vi "overlay_axis_particle(subVI).vi"(8 "error in (no error)":errorcluster, 9 "filtred & calibrated image":T1, 10 "view image":T1) -> (0 "error out":errorcluster, 1 "Particle Reports (Real-World)":T2(array[cluster]) {"Orientation" format="%.2f"; "Dimensions"."Height" format="%.2f"; "Dimensions"."Width" format="%.2f"; "Center of Mass"."Y" format="%.2f"; "Center of Mass"."X" format="%.2f"; "Bounding Rect"."Bottom" format="%.2f"; "Bounding Rect"."Right" format="%.2f"; "Bounding Rect"."Top" format="%.2f"; "Bounding Rect"."Left" format="%.2f"; "Number of Holes" format="%.2f"; "Area" format="%.2f"}, 2 "number of particle":i32, 3 "Image Out":T1)   [LabVIEW 2020]
uses:
  <vilib>/vision/Image Controls.llb/IMAQ Image.ctl
  <vilib>/vision/NI_Vision_Development_Module.lvlib
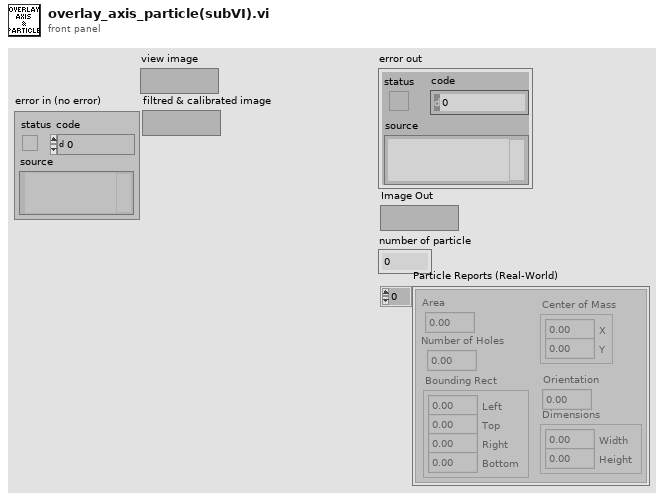
[diagram p1: front panel]
types:
  T1 = typedef "IMAQ Image.ctl" = refnum<image>
  T2 = cluster{"Area":dbl, "Number of Holes":dbl, "Bounding Rect":cluster{"Left":dbl, "Top":dbl, "Right":dbl, "Bottom":dbl}, "Center of Mass":cluster{"X":dbl, "Y":dbl}, "Orientation":dbl, "Dimensions":cluster{"Width":dbl, "Height":dbl}}[]
  T3 = cluster{"Origin Pixel":cluster{"X":sgl, "Y":sgl}, "Angle Relative to Horizontal (deg)":sgl, "Axis Reference":u32}
  T4 = cluster{"Origin Pixel":cluster{"X":sgl, "Y":sgl}, "Angle Relative to Horizontal (deg)":sgl, "X Axis Pixel":cluster{"X":sgl, "Y":sgl}, "Axis Reference":u32}
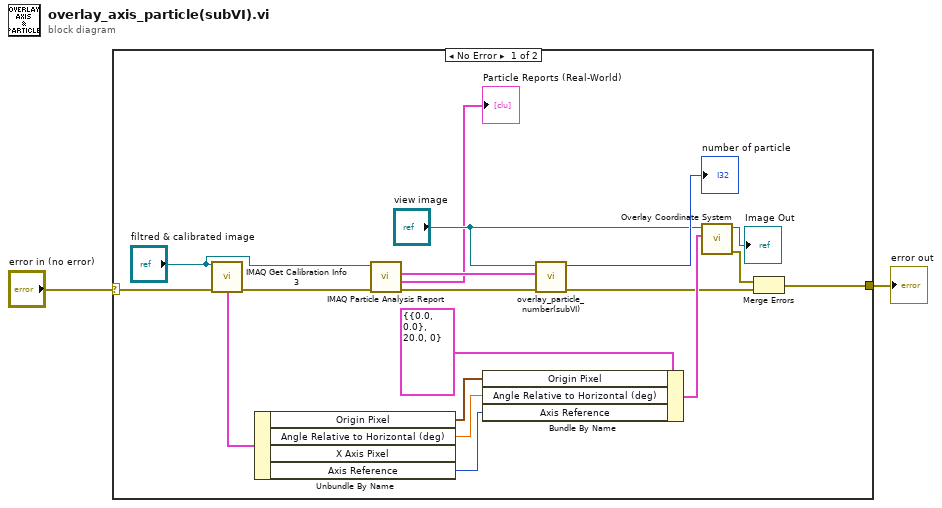
[diagram p0: block diagram]
diagram:
  n1 = case shown="No Error" "error in (no error)" {
    selector: "error in (no error)" -> [w13 w21]
    tunnel: [w15 w21] -> w2
    frame No Error {
      n2 = call "IMAQ Get Calibration Info 3"("Calibration Template Image"="filtred & calibrated image", "error in (no error)"=w13) -> ("Calibration Axis Info"=w8:T4, "error out"=w11:errorcluster)  [unwired: 5 in, 7 out]
      n3 = Unbundle By Name(w8) -> ("Origin Pixel"=w6:cluster{"X":sgl, "Y":sgl}, "Angle Relative to Horizontal (deg)"=w5:sgl, "Axis Reference"=w7:u32)  [unwired: 1 out]
      n4 = call "IMAQ Particle Analysis Report"("error in (no error)"=w11, "Image"="filtred & calibrated image") -> ("error out"=w10:errorcluster, "Particle Reports (Real-World)"=→"Particle Reports (Real-World)":T2, "Particle Reports (Pixels)"=w9:T2)  [unwired: 4 in, 3 out]
      n5 = Bundle By Name(cluster=T3 {"Origin Pixel"={"X"=0.0, "Y"=0.0}, "Angle Relative to Horizontal (deg)"=20.0, "Axis Reference"=0} ("Calibration Axis Info"), "Origin Pixel"=w6, "Angle Relative to Horizontal (deg)"=w5, "Axis Reference"=w7) -> (w19:T3)
      n6 = call "overlay_particle_number(subVI).vi"("error in (no error)"=w10, "Particle Reports (Pixels)"=w9, "Image"="view image") -> ("error out"=w17:errorcluster, "number of particle"=→"number of particle":i32)  [unwired: 7 in]
      n7 = call "Overlay Coordinate System.vi"("Calibration Axis Info"=w19, "Image"="view image") -> ("error out"=w16:errorcluster, "Image Out"=→"Image Out":T1)  [unwired: 8 in]
      n8 = Merge Errors(w16, w17) -> (w15:errorcluster)
    }
    frame Error {
    }
  }
  "error out" <- w2
